vi "System_Time_in_Seconds.vi"() -> (0 "Current Time (s)":dbl)   [LabVIEW 2010]
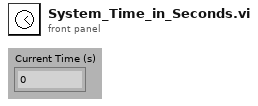
[diagram p1: front panel]
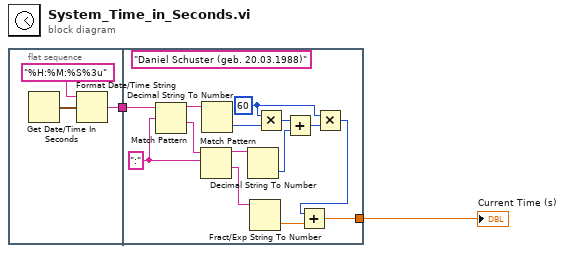
[diagram p0: block diagram]
diagram:
  (unwired) "Daniel Schuster (geb. 20.03.1988)"
  n1 = flat-sequence {
    tunnel: [w3] -> w2
    tunnel: [w7] -> w1
    tunnel: w2 -> [w6]
    frame #0 {
      n2 = Get Date/Time In Seconds() -> (seconds since 1Jan1904=w4:timestamp)
      n3 = Format Date/Time String(time format string (%c)="%H:%M:%S%3u", seconds (now)=w4) -> (date/time string=w3:string)  [unwired: 1 in]
    }
    frame #1 {
      w9 = 60
      w18 = ":"
      n4 = Match Pattern(string=w6, regular expression=w18) -> (before substring=w17:string, after substring=w19:string)  [unwired: 1 in, 2 out]
      n5 = Match Pattern(string=w19, regular expression=w18) -> (before substring=w16:string, after substring=w15:string)  [unwired: 1 in, 2 out]
      n6 = Decimal String To Number(string=w17) -> (number=w14:i32)  [unwired: 2 in, 1 out]
      n7 = Decimal String To Number(string=w16) -> (number=w8:i32)  [unwired: 2 in, 1 out]
      n8 = Fract/Exp String To Number(string=w15) -> (number=w10:dbl)  [unwired: 3 in, 1 out]
      n9 = Multiply(x=w9, y=w14) -> (x*y=w13:i32)
      n10 = Add(x=w13, y=w8) -> (x+y=w12:i32)
      n11 = Multiply(x=w9, y=w12) -> (x*y=w11:i32)
      n12 = Add(x=w11, y=w10) -> (x+y=w7:dbl)
    }
  }
  "Current Time (s)" <- w1
